vi "photo_encoder_sub.vi"(10 "reference":refnum<vi>, 11 "Digital in":refnum<vi>) -> ()   [LabVIEW 2014]
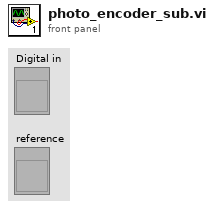
[diagram p1: front panel]
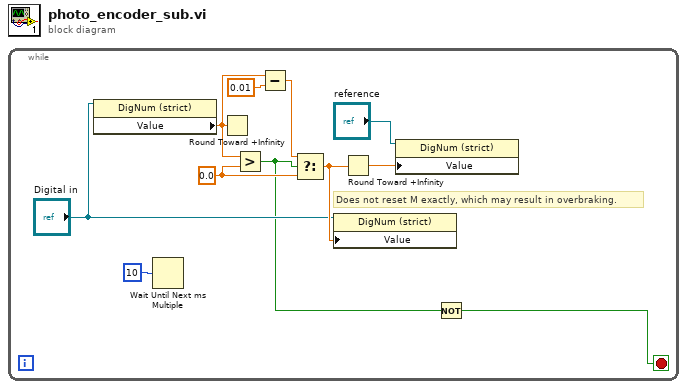
[diagram p0: block diagram]
diagram:
  n1 = while {
    stop <- w2 stop-if-true
    w8 = 0.0 ("y")
    # "Does not reset M exactly, which may result in overbraking."
    n2 = property class="DigNum (strict)"(reference="Digital in") -> ("Value"=w10:dbl)  [unwired: 1 in, 2 out]
    n3 = Wait Until Next ms Multiple(millisecond multiple=u32 10) -> ()  [unwired: 1 out]
    n4 = Round Toward +Infinity(x=w10) -> ()  [unwired: 1 out]
    n5 = Greater?(x=w10, y=w8) -> (0:w3:bool)
    n6 = Subtract(x=w10, y=0.01) -> (x-y=w9:dbl)
    n7 = Select(t=w9, s=w3, f=w8) -> (s? t:f=w11:dbl)
    n8 = property class="DigNum (strict)"(reference="Digital in", "Value"=w11) -> ()  [unwired: 1 in, 2 out]
    n9 = Round Toward +Infinity(x=w11) -> (ceil(x): smallest int >= x=w7:dbl)
    n10 = property class="DigNum (strict)"(reference="reference", "Value"=w7) -> ()  [unwired: 1 in, 2 out]
    n11 = Not(x=w3) -> (.not. x?=w2:bool)
  }
